vi "util_get_change_in.vi"(7 "references":T1, 8 "error in (no error)":errorcluster, 10 "timeout":i32, 11 "ignore_previous":bool) -> (0 "error out":errorcluster, 2 "data":variant, 3 "change?":bool)   [LabVIEW 2015, in "repub-dvr_nre.lvlib"]
uses:
  repub-dvr_nre.lvlib
  public/_controls/references.ctl
  _controls/input.ctl
  _controls/input_command.ctl
  _controls/output.ctl
  _controls/data.ctl
  public/_controls/configuration.ctl
  public/_controls/change.ctl
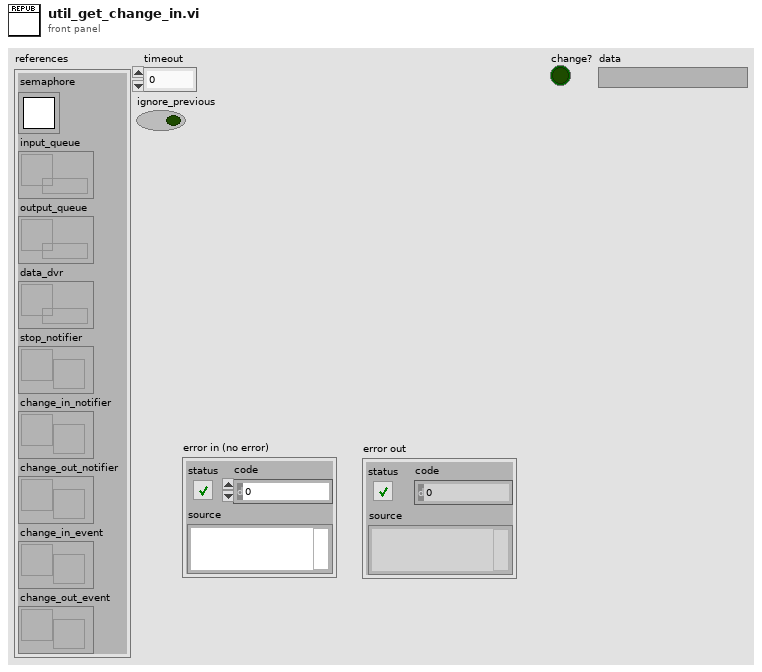
[diagram p1: front panel]
types:
  T1 = typedef "repub-dvr_nre.lvlib/references.ctl" = cluster{"semaphore":T2, "input_queue":refnum<queue>, "output_queue":refnum<queue>, "data_dvr":refnum<data-value>, "stop_notifier":refnum<notifier>, "change_in_notifier":refnum<notifier>, "change_out_notifier":refnum<notifier>, "change_in_event":refnum<user-event>, "change_out_event":refnum<user-event>}
  T2 = typedef "Semaphore RefNum" = refnum<k1>
  T3 = typedef "repub-dvr_nre.lvlib/change.ctl" = cluster{"data_changed":bool, "data":variant}
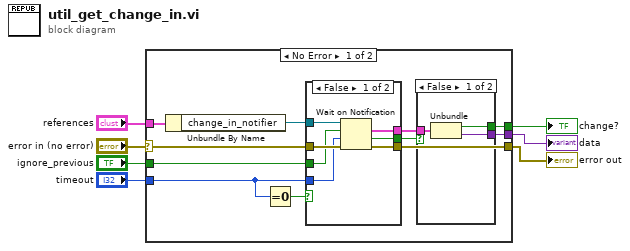
[diagram p0: block diagram]
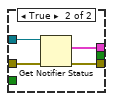
[diagram p3: hidden frame]
diagram:
  n1 = case shown="No Error" "error in (no error)" {
    selector: "error in (no error)" -> [w16 w33]
    tunnel: [w12 w33] -> w6
    tunnel: "references" -> [w18 _]
    tunnel: "timeout" -> [w15 _]
    tunnel: "ignore_previous" -> [w13 _]
    tunnel: [w9 _] -> w2
    tunnel: [w8 _] -> w1
    frame No Error {
      n2 = Unbundle By Name(w18) -> ("change_in_notifier"=w17:refnum<notifier>)
      n3 = Equal To 0?(x=w15) -> (x = 0?=w14:bool)
      n4 = case shown="False" w14 {
        tunnel: w17 -> [w28 w32]
        tunnel: w16 -> [w27 w31]
        tunnel: w15 -> [w26 _]
        tunnel: w13 -> [w25 _]
        tunnel: [w24 w30] -> w10
        tunnel: [w23 _] -> w11
        tunnel: [w22 w29] -> w12
        frame False {
          n5 = Wait on Notification(notifier=w28, ignore previous (F)=w25, timeout in ms (-1)=w26, error in (no error)=w27) -> (notification=w24:T3, timed out?=w23:bool, error out=w22:errorcluster)  [unwired: 1 out]
        }
        frame True {
          n6 = Get Notifier Status(notifier=w32, error in (no error)=w31) -> (current notification=w30:T3, error out=w29:errorcluster)  [unwired: 3 out]
        }
      }
      n7 = case shown="False" w11 {
        tunnel: w10 -> [w21 _]
        tunnel: [w20 _] -> w9
        tunnel: [w19 _] -> w8
        frame False {
          n8 = Unbundle(w21) -> ("data_changed"=w20:bool, "data"=w19:variant)
        }
        frame True {
        }
      }
    }
    frame Error {
    }
  }
  "error out" <- w6
  "change?" <- w2
  "data" <- w1
